vi "prompt user for configuration.vi"(8 "error in (no error)":errorcluster) -> (0 "error out":errorcluster, 2 "cancelled":bool, 3 "selected path":path)   [LabVIEW 2024, in "DSF System Explorer.lvlib"]
uses:
  DSF System Explorer.lvlib
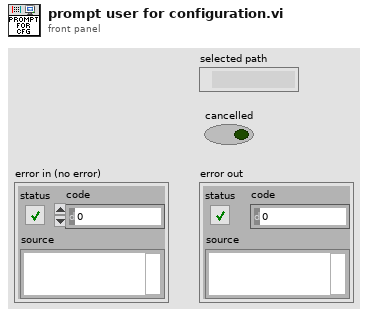
[diagram p1: front panel]
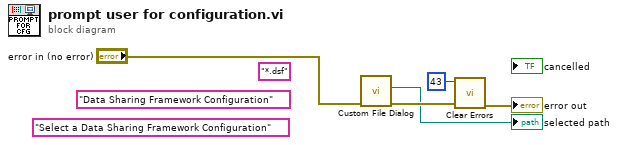
[diagram p0: block diagram]
diagram:
  (unwired) "Select a Data Sharing Framework Configuration" ("prompt")
  (unwired) "Data Sharing Framework Configuration" ("pattern label")
  (unwired) "*.dsf" ("pattern (all files)")
  n1 = call "Custom File Dialog.vi"("error in (no error)"="error in (no error)") -> ("error out"=w2:errorcluster, "path out"=→"selected path":path)  [unwired: 9 in]
  n2 = call <vilib>:"Clear Errors.vi"("error in (no error)"=w2, "specific error code to clear (0: all)"=43) -> ("error out"=→"error out":errorcluster)  [unwired: 4 in, 1 out]
